vi "TCP seq handler.vi"   [LabVIEW 2021]
uses:
  TCP states.ctl
types:
  T1 = typedef "TCP states.ctl" = string
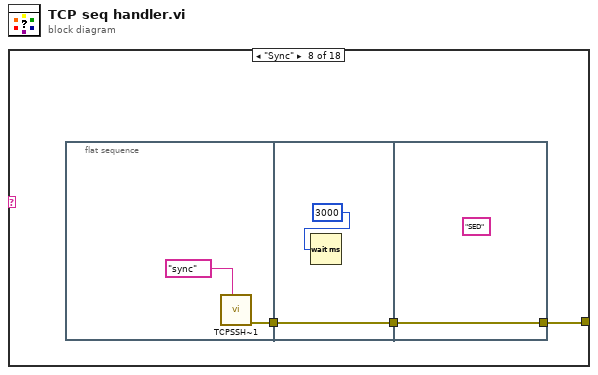
[diagram p0: block diagram]
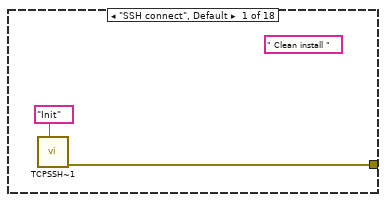
[diagram p2: hidden frame]
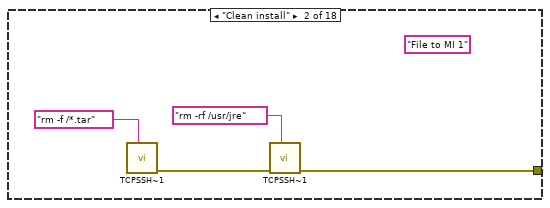
[diagram p3: hidden frame]
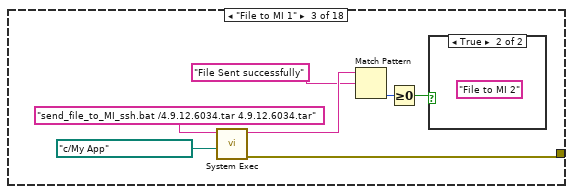
[diagram p4: hidden frame]
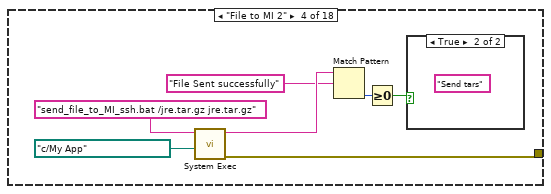
[diagram p6: hidden frame]
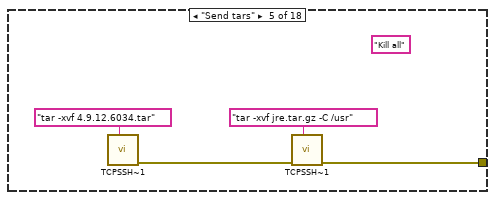
[diagram p8: hidden frame]
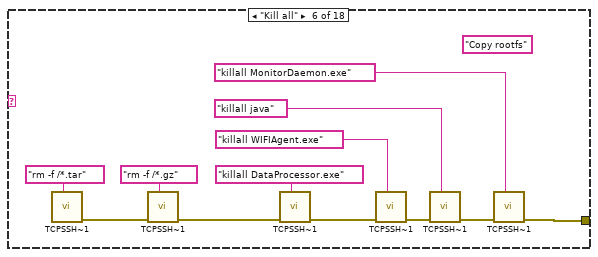
[diagram p9: hidden frame]
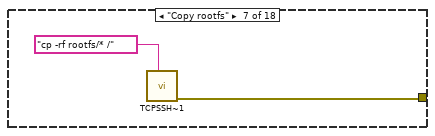
[diagram p10: hidden frame]
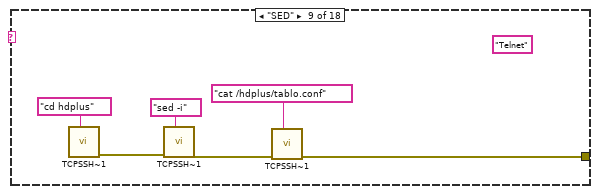
[diagram p11: hidden frame]
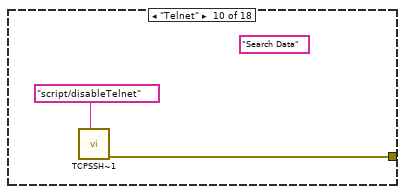
[diagram p12: hidden frame]
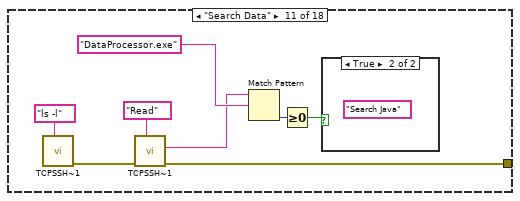
[diagram p13: hidden frame]
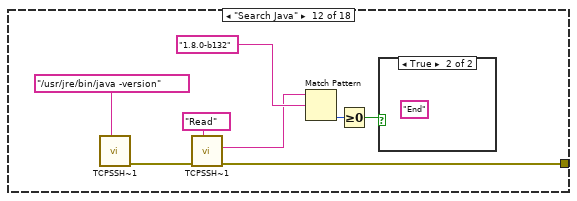
[diagram p15: hidden frame]
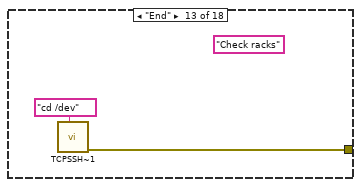
[diagram p17: hidden frame]
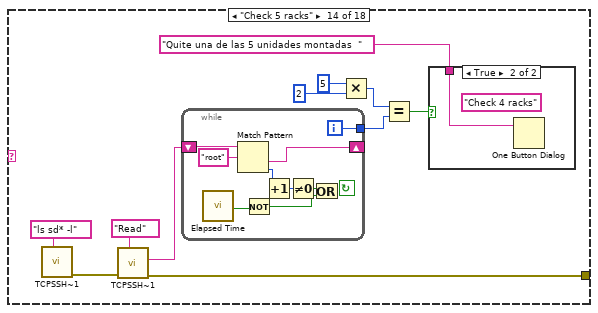
[diagram p18: hidden frame]
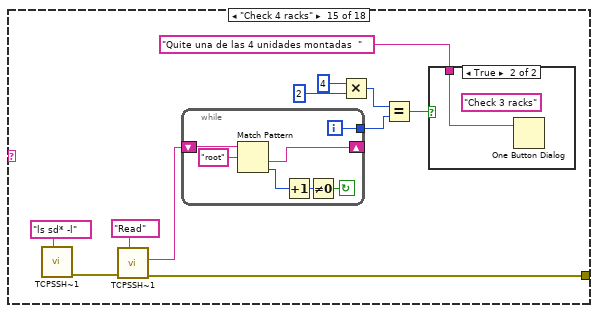
[diagram p20: hidden frame]
diagram:
  n1 = case shown="\"Sync\"" {
    selector: _ -> [_ _ _ _ _ _ _ _ _ _ _ _ _ _ _ _ _ _]
    tunnel: [w1 w3 w13 w20 w21 w26 w37 w41 w47 w53 w55 w63 w71 w74 w95 w114 w133 w151] -> _
    frame "SSH connect", Default {
      (unwired) " Clean install "
      n2 = call "TCPSSH~1.VI"("States"=T1 "Init") -> ("Error  Out"=w1:errorcluster)  [unwired: 8 in, 1 out]
    }
    frame "Clean install" {
      (unwired) "File to MI 1"
      n3 = call "TCPSSH~1.VI"("States"=T1 "rm -f /*.tar") -> ("Error  Out"=w4:errorcluster)  [unwired: 8 in, 1 out]
      n4 = call "TCPSSH~1.VI"("States"=T1 "rm -rf /usr/jre", "Error In"=w4) -> ("Error  Out"=w3:errorcluster)  [unwired: 7 in, 1 out]
    }
    frame "File to MI 1" {
      n5 = call <vilib>:"System Exec.vi"("working directory"=path "c:/My App", "command line"="send_file_to_MI_ssh.bat /4.9.12.6034.tar 4.9.12.6034.tar") -> ("error out"=w13:errorcluster, "standard output"=w10:string)  [unwired: 6 in, 2 out]
      n6 = Match Pattern(string=w10, regular expression="File Sent successfully") -> (offset past match=w8:i32)  [unwired: 1 in, 3 out]
      n7 = Greater Or Equal To 0?(x=w8) -> (x >= 0?=w7:bool)
      n8 = case shown="True" w7 {
        frame False {
        }
        frame True {
          (unwired) "File to MI 2"
        }
      }
    }
    frame "File to MI 2" {
      n9 = call <vilib>:"System Exec.vi"("working directory"=path "c:/My App", "command line"="send_file_to_MI_ssh.bat /jre.tar.gz jre.tar.gz") -> ("error out"=w20:errorcluster, "standard output"=w17:string)  [unwired: 6 in, 2 out]
      n10 = Match Pattern(string=w17, regular expression="File Sent successfully") -> (offset past match=w15:i32)  [unwired: 1 in, 3 out]
      n11 = Greater Or Equal To 0?(x=w15) -> (x >= 0?=w14:bool)
      n12 = case shown="True" w14 {
        frame False {
        }
        frame True {
          (unwired) "Send tars"
        }
      }
    }
    frame "Send tars" {
      (unwired) "Kill all"
      n13 = call "TCPSSH~1.VI"("States"=T1 "tar -xvf 4.9.12.6034.tar") -> ("Error  Out"=w22:errorcluster)  [unwired: 8 in, 1 out]
      n14 = call "TCPSSH~1.VI"("States"=T1 "tar -xvf jre.tar.gz -C /usr", "Error In"=w22) -> ("Error  Out"=w21:errorcluster)  [unwired: 7 in, 1 out]
    }
    frame "Kill all" {
      (unwired) "Copy rootfs"
      n15 = call "TCPSSH~1.VI"("States"=T1 "rm -f /*.tar") -> ("Error  Out"=w34:errorcluster)  [unwired: 8 in, 1 out]
      n16 = call "TCPSSH~1.VI"("States"=T1 "rm -f /*.gz", "Error In"=w34) -> ("Error  Out"=w32:errorcluster)  [unwired: 7 in, 1 out]
      n17 = call "TCPSSH~1.VI"("States"=T1 "killall DataProcessor.exe", "Error In"=w32) -> ("Error  Out"=w31:errorcluster)  [unwired: 7 in, 1 out]
      n18 = call "TCPSSH~1.VI"("States"=T1 "killall WIFIAgent.exe", "Error In"=w31) -> ("Error  Out"=w29:errorcluster)  [unwired: 7 in, 1 out]
      n19 = call "TCPSSH~1.VI"("States"=T1 "killall java", "Error In"=w29) -> ("Error  Out"=w27:errorcluster)  [unwired: 7 in, 1 out]
      n20 = call "TCPSSH~1.VI"("States"=T1 "killall MonitorDaemon.exe", "Error In"=w27) -> ("Error  Out"=w26:errorcluster)  [unwired: 7 in, 1 out]
    }
    frame "Copy rootfs" {
      n21 = call "TCPSSH~1.VI"("States"=T1 "cp -rf rootfs/* /") -> ("Error  Out"=w37:errorcluster)  [unwired: 8 in, 1 out]
    }
    frame "Sync" {
      n22 = flat-sequence {
        tunnel: [w42] -> w40
        tunnel: w40 -> [w45]
        tunnel: [w45] -> w39
        tunnel: [w46] -> w41
        tunnel: w39 -> [w46]
        frame #0 {
          n23 = call "TCPSSH~1.VI"("States"=T1 "sync") -> ("Error  Out"=w42:errorcluster)  [unwired: 8 in, 1 out]
        }
        frame #1 {
          n24 = Wait (ms)(milliseconds to wait=u32 3000) -> ()  [unwired: 1 out]
        }
        frame #2 {
          (unwired) "SED"
        }
      }
    }
    frame "SED" {
      (unwired) "Telnet"
      n25 = call "TCPSSH~1.VI"("States"=T1 "cd hdplus") -> ("Error  Out"=w50:errorcluster)  [unwired: 8 in, 1 out]
      n26 = call "TCPSSH~1.VI"("States"=T1 "sed -i", "Error In"=w50) -> ("Error  Out"=w48:errorcluster)  [unwired: 7 in, 1 out]
      n27 = call "TCPSSH~1.VI"("States"=T1 "cat /hdplus/tablo.conf", "Error In"=w48) -> ("Error  Out"=w47:errorcluster)  [unwired: 7 in, 1 out]
    }
    frame "Telnet" {
      (unwired) "Search Data"
      n28 = call "TCPSSH~1.VI"("States"=T1 "script/disableTelnet") -> ("Error  Out"=w53:errorcluster)  [unwired: 8 in, 1 out]
    }
    frame "Search Data" {
      n29 = call "TCPSSH~1.VI"("States"=T1 "ls -l") -> ("Error  Out"=w61:errorcluster)  [unwired: 8 in, 1 out]
      n30 = call "TCPSSH~1.VI"("States"=T1 "Read", "Error In"=w61) -> ("Error  Out"=w55:errorcluster, "Response"=w56:string)  [unwired: 7 in]
      n31 = Match Pattern(string=w56, regular expression="DataProcessor.exe") -> (offset past match=w59:i32)  [unwired: 1 in, 3 out]
      n32 = Greater Or Equal To 0?(x=w59) -> (x >= 0?=w58:bool)
      n33 = case shown="True" w58 {
        frame False {
        }
        frame True {
          (unwired) "Search Java"
        }
      }
    }
    frame "Search Java" {
      n34 = call "TCPSSH~1.VI"("States"=T1 "/usr/jre/bin/java -version") -> ("Error  Out"=w69:errorcluster)  [unwired: 8 in, 1 out]
      n35 = call "TCPSSH~1.VI"("States"=T1 "Read", "Error In"=w69) -> ("Error  Out"=w63:errorcluster, "Response"=w64:string)  [unwired: 7 in]
      n36 = Match Pattern(string=w64, regular expression="1.8.0-b132") -> (offset past match=w67:i32)  [unwired: 1 in, 3 out]
      n37 = Greater Or Equal To 0?(x=w67) -> (x >= 0?=w66:bool)
      n38 = case shown="True" w66 {
        frame False {
        }
        frame True {
          (unwired) "End"
        }
      }
    }
    frame "End" {
      (unwired) "Check racks"
      n39 = call "TCPSSH~1.VI"("States"=T1 "cd /dev") -> ("Error  Out"=w71:errorcluster)  [unwired: 8 in, 1 out]
    }
    frame "Check 5 racks" {
      n40 = call "TCPSSH~1.VI"("States"=T1 "ls sd* -l") -> ("Error  Out"=w81:errorcluster)  [unwired: 8 in, 1 out]
      n41 = call "TCPSSH~1.VI"("States"=T1 "Read", "Error In"=w81) -> ("Error  Out"=w74:errorcluster, "Response"=w80:string)  [unwired: 7 in]
      n42 = while {
        shift-right: [w91] -> _
        shift-left: w80 -> [w93]
        tunnel: [w88] -> w76
        i -> [w88]
        stop <- _ continue-if-true
        n43 = call "Elapsed Time"() -> ("Time has Elapsed"=w87:bool)  [unwired: 12 in, 7 out]
        n44 = Match Pattern(string=w93, regular expression="root") -> (after substring=w91:string, offset past match=w90:i32)  [unwired: 1 in, 2 out]
        n45 = Not(x=w87) -> (.not. x?=w86:bool)
        n46 = Increment(x=w90) -> (x+1=w89:i32)
        n47 = Not Equal To 0?(x=w89) -> (x != 0?=w85:bool)
        n48 = Or(x=w85, y=w86) -> ()  [unwired: 1 out]
      }
      n49 = Multiply(x=5, y=2) -> (x*y=w77:i32)
      n50 = Equal?(x=w77, y=w76) -> (x = y?=w75:bool)
      n51 = case shown="True" w75 {
        tunnel: "Quite una de las 5 unidades montadas  " ("message") -> [_ w84]
        frame False {
        }
        frame True {
          (unwired) "Check 4 racks"
          n52 = One Button Dialog(message=w84) -> ()  [unwired: 1 in, 1 out]
        }
      }
    }
    frame "Check 4 racks" {
      n53 = call "TCPSSH~1.VI"("States"=T1 "ls sd* -l") -> ("Error  Out"=w102:errorcluster)  [unwired: 8 in, 1 out]
      n54 = call "TCPSSH~1.VI"("States"=T1 "Read", "Error In"=w102) -> ("Error  Out"=w95:errorcluster, "Response"=w101:string)  [unwired: 7 in]
      n55 = while {
        shift-right: [w110] -> _
        shift-left: w101 -> [w112]
        tunnel: [w106] -> w97
        i -> [w106]
        stop <- w107 continue-if-true
        n56 = Match Pattern(string=w112, regular expression="root") -> (after substring=w110:string, offset past match=w109:i32)  [unwired: 1 in, 2 out]
        n57 = Increment(x=w109) -> (x+1=w108:i32)
        n58 = Not Equal To 0?(x=w108) -> (x != 0?=w107:bool)
      }
      n59 = Multiply(x=4, y=2) -> (x*y=w98:i32)
      n60 = Equal?(x=w98, y=w97) -> (x = y?=w96:bool)
      n61 = case shown="True" w96 {
        tunnel: "Quite una de las 4 unidades montadas  " ("message") -> [_ w105]
        frame False {
        }
        frame True {
          (unwired) "Check 3 racks"
          n62 = One Button Dialog(message=w105) -> ()  [unwired: 1 in, 1 out]
        }
      }
    }
    frame "Check 3 racks" {
      n63 = call "TCPSSH~1.VI"("States"=T1 "ls sd* -l") -> ("Error  Out"=w121:errorcluster)  [unwired: 8 in, 1 out]
      n64 = call "TCPSSH~1.VI"("States"=T1 "Read", "Error In"=w121) -> ("Error  Out"=w114:errorcluster, "Response"=w120:string)  [unwired: 7 in]
      n65 = while {
        shift-right: [w129] -> _
        shift-left: w120 -> [w131]
        tunnel: [w125] -> w116
        i -> [w125]
        stop <- w126 continue-if-true
        n66 = Match Pattern(string=w131, regular expression="root") -> (after substring=w129:string, offset past match=w128:i32)  [unwired: 1 in, 2 out]
        n67 = Increment(x=w128) -> (x+1=w127:i32)
        n68 = Not Equal To 0?(x=w127) -> (x != 0?=w126:bool)
      }
      n69 = Multiply(x=3, y=2) -> (x*y=w117:i32)
      n70 = Equal?(x=w117, y=w116) -> (x = y?=w115:bool)
      n71 = case shown="True" w115 {
        tunnel: "Quite una de las 3 unidades montadas  " ("message") -> [_ w124]
        frame False {
        }
        frame True {
          (unwired) "Check 2 racks"
          n72 = One Button Dialog(message=w124) -> ()  [unwired: 1 in, 1 out]
        }
      }
    }
    frame "Check 2 racks" {
      n73 = call "TCPSSH~1.VI"("States"=T1 "ls sd* -l") -> ("Error  Out"=w140:errorcluster)  [unwired: 8 in, 1 out]
      n74 = call "TCPSSH~1.VI"("States"=T1 "Read", "Error In"=w140) -> ("Error  Out"=w133:errorcluster, "Response"=w139:string)  [unwired: 7 in]
      n75 = while {
        shift-right: [w148] -> _
        shift-left: w139 -> [w150]
        tunnel: [w144] -> w135
        i -> [w144]
        stop <- w145 continue-if-true
        n76 = Match Pattern(string=w150, regular expression="root") -> (after substring=w148:string, offset past match=w147:i32)  [unwired: 1 in, 2 out]
        n77 = Increment(x=w147) -> (x+1=w146:i32)
        n78 = Not Equal To 0?(x=w146) -> (x != 0?=w145:bool)
      }
      n79 = Multiply(x=2, y=2) -> (x*y=w136:i32)
      n80 = Equal?(x=w136, y=w135) -> (x = y?=w134:bool)
      n81 = case shown="True" w134 {
        tunnel: "Quite una de las 2 unidades montadas  " ("message") -> [_ w143]
        frame False {
        }
        frame True {
          (unwired) "Check 1 racks"
          n82 = One Button Dialog(message=w143) -> ()  [unwired: 1 in, 1 out]
        }
      }
    }
    frame "Check 1 racks" {
      n83 = call "TCPSSH~1.VI"("States"=T1 "ls sd* -l") -> ("Error  Out"=w158:errorcluster)  [unwired: 8 in, 1 out]
      n84 = call "TCPSSH~1.VI"("States"=T1 "Read", "Error In"=w158) -> ("Error  Out"=w151:errorcluster, "Response"=w157:string)  [unwired: 7 in]
      n85 = while {
        shift-right: [w166] -> _
        shift-left: w157 -> [w168]
        tunnel: [w162] -> w153
        i -> [w162]
        stop <- w163 continue-if-true
        n86 = Match Pattern(string=w168, regular expression="root") -> (after substring=w166:string, offset past match=w165:i32)  [unwired: 1 in, 2 out]
        n87 = Increment(x=w165) -> (x+1=w164:i32)
        n88 = Not Equal To 0?(x=w164) -> (x != 0?=w163:bool)
      }
      n89 = Multiply(x=1, y=2) -> (x*y=w154:i32)
      n90 = Equal?(x=w154, y=w153) -> (x = y?=w152:bool)
      n91 = case shown="True" w152 {
        frame False {
        }
        frame True {
          n92 = One Button Dialog(message="Completado!") -> ()  [unwired: 1 in, 1 out]
        }
      }
    }
  }
